vi "FLIM UI example.vi"(8 "error in (no error)":errorcluster) -> (0 "error out":errorcluster)   [LabVIEW 2014]
uses:
  typedefs/ScanControl_typedef.ctl
  typedefs/ScannerCommands_typedef.ctl
  typedefs/Command Queue element typedef.ctl
  SwabianInstruments.TimeTagger
panel:
  in  "Demo":bool caption="Enable demo signal"
  in  "Conditional Filter":bool
  in  "StopScan":bool
  out "Frame Progress":u8(slide) scale=0.0..100.0
  in  "scan_tagger":bool
  in  "TTs_found":i32(listbox)=-1 caption="Taggers found"
  out "Scanning":bool
  out "error msg":string caption="Error message"
  in  "Scan range":T1={"x-axis"={"start"=0.0, "num"=150, "step"=1.0}, "y-axis"={"start"=0.0, "num"=100, "step"=1.0}}
  out "Histogram at location":T2(graph)
  out "Intensity image":sgl[][](graph)
  in  "frame_start":enum32{"None", "Channel"}(tab) caption="Frame start marker"
  in  "FRAME_BEGIN_CH":i32
  in  "averages per frame":u32=1 min=1 step=1
  in  "frames to acquire":u32=1 step=1
  in  "n_bins":i32=100
  in  "Binwidth":dbl[unit]=1e-11
  in  "StartScan":bool
  in  "close":bool
  out "Time Tagger":string caption="Connected Time Tagger:"
  in  "Connect":bool
  in  "Pixel end marker":T3(tab)
  in  "Pixel duration time":dbl[unit] format="%^.3e"
  in  "PIXEL_END_CH":i32=-3
  in  "PIXEL_BEGIN_CH":i32=3
  in  "DET_CH":i32=2
  in  "LASER_CH":i32=1
  # "DESCRIPTION\nThis VI is an example.  It implements FLIM data acquisition part only and demonstrates how\nto use Flim class provided with the Time Tagger software.\n\nIt is designed as a template and a reasonybly good starting point for development of your \nown FLIM experiment control program.\n\nThis example provides demo signal that you can enable for testing purpose. The expected\nscan result with a demo sognal is a checkerboard-like intensity image."
  # "Do not use frame start marker.\nFrame begins automatcally."
  # "Pulse duration defines \npixel integration time"
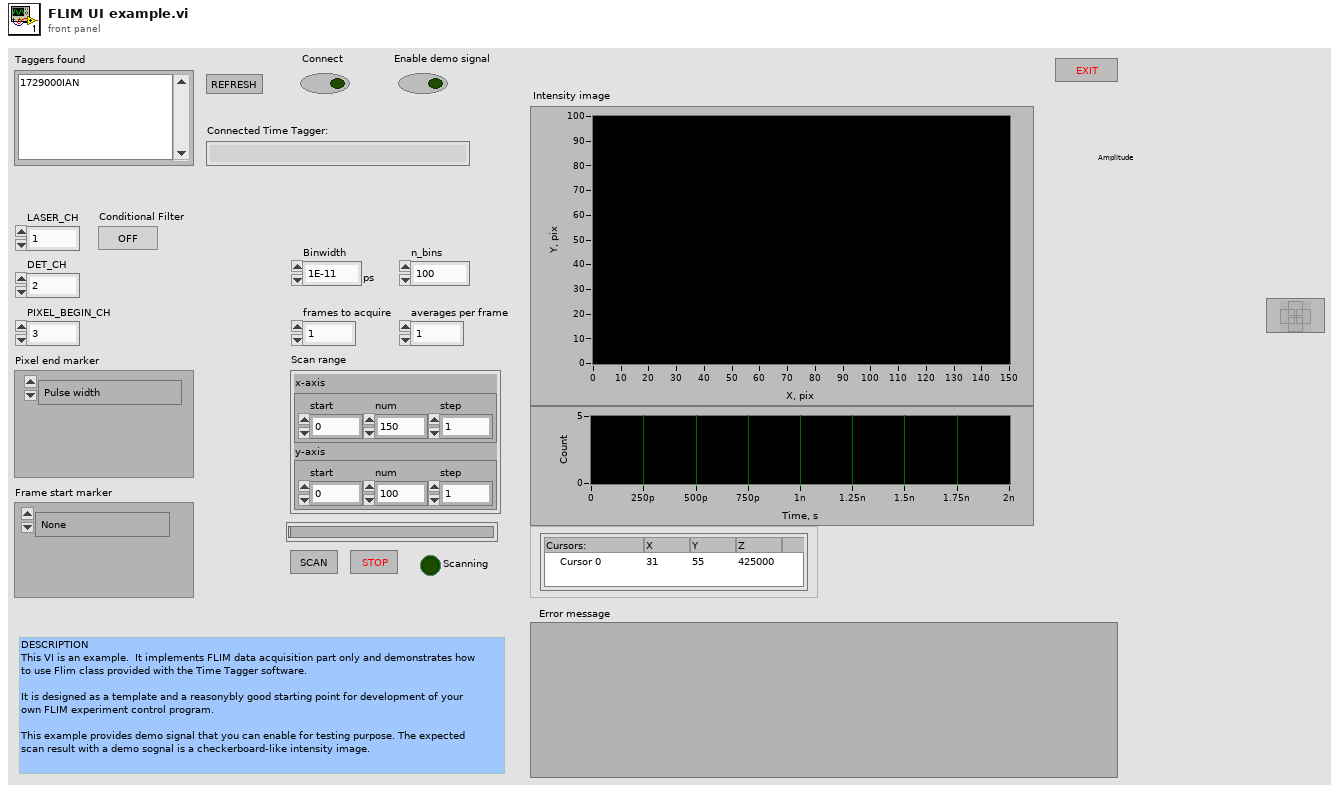
[diagram p1: front panel]
types:
  T1 = typedef "ScanControl_typedef.ctl" = cluster{"x-axis":cluster{"start":dbl, "num":u32, "step":dbl}, "y-axis":cluster{"start":dbl, "num":u32, "step":dbl}}
  T2 = cluster{dbl, "Binwidth":dbl[unit], "getHistograms":u32[]}
  T3 = enum32{"Pulse width", "Begin+duration", "End channel"}
  T4 = typedef "Command Queue element typedef.ctl" = cluster{"CMD":T5, "Scan range":T1}
  T5 = typedef "ScannerCommands_typedef.ctl" = enum16{"Do nothing", "Start Scan", "Stop Scan"}
  T6 = cluster{"TTlib":refnum<k24>, "tagger":refnum<k24>, "flim":refnum<k24>, "pixel_end_vch":refnum<k24>, "flim_frame":refnum<k24>, "Scan range":T1, "cmd_queue":refnum<queue>}
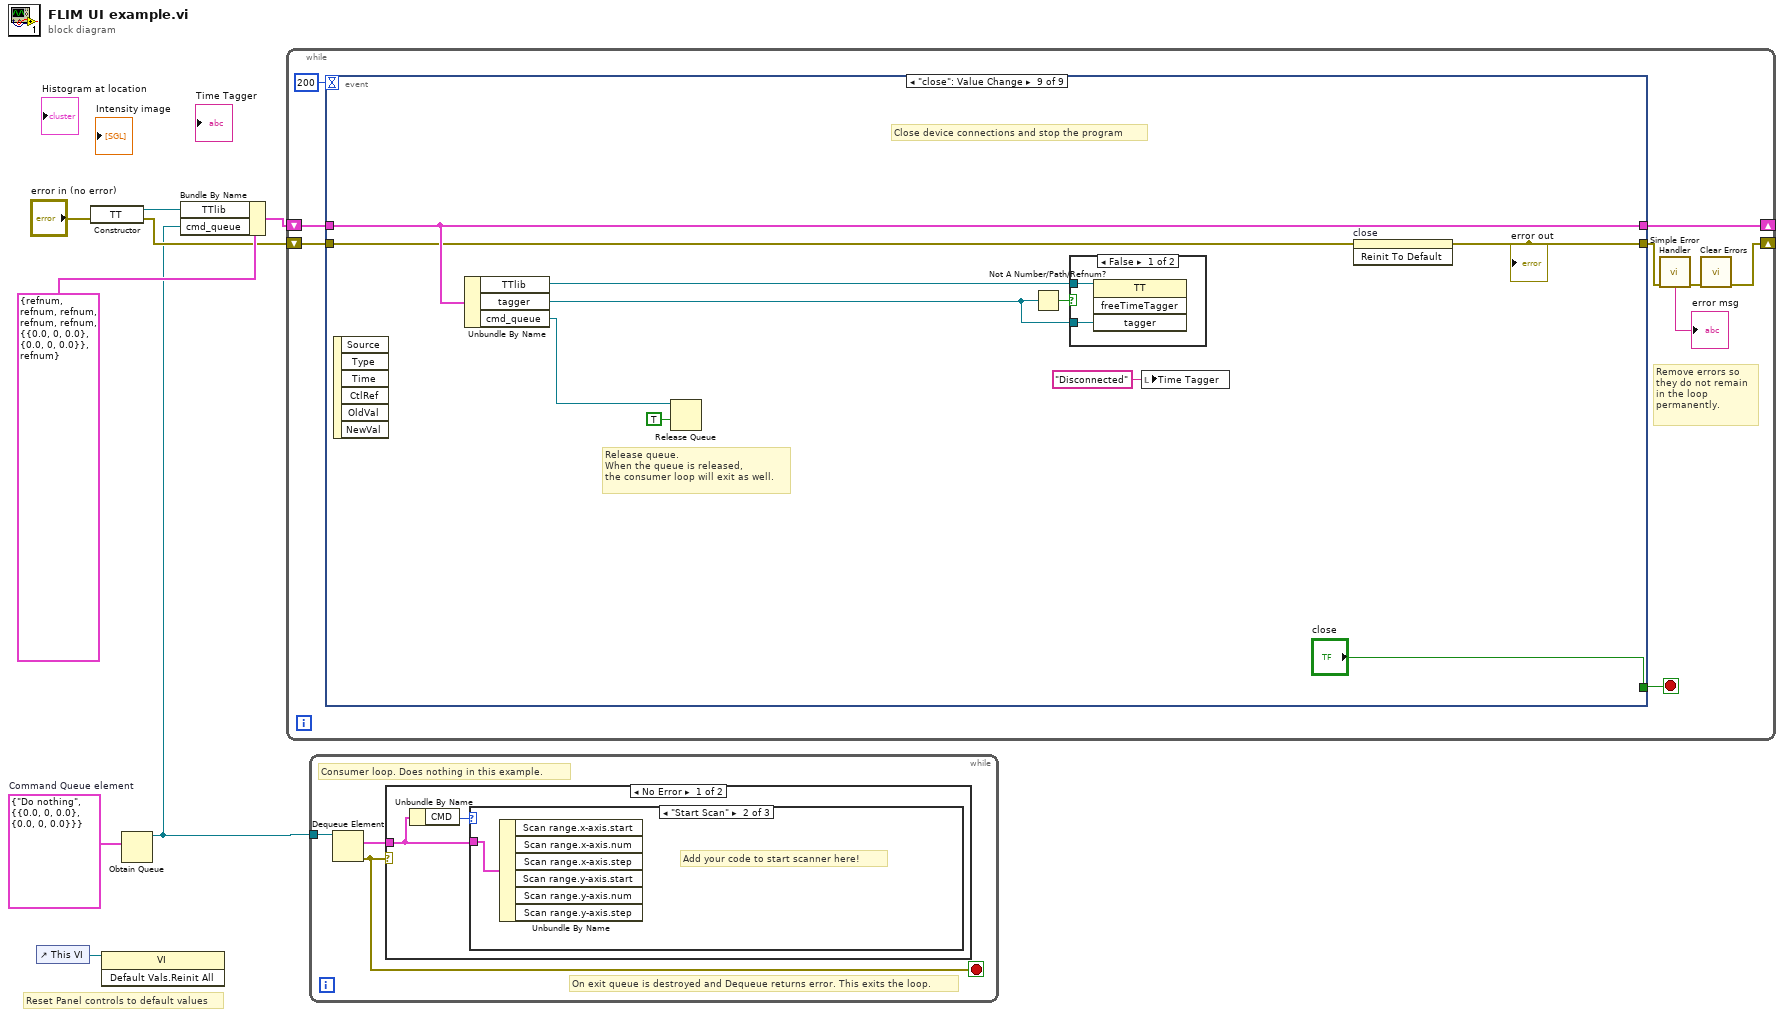
[diagram p0: block diagram]
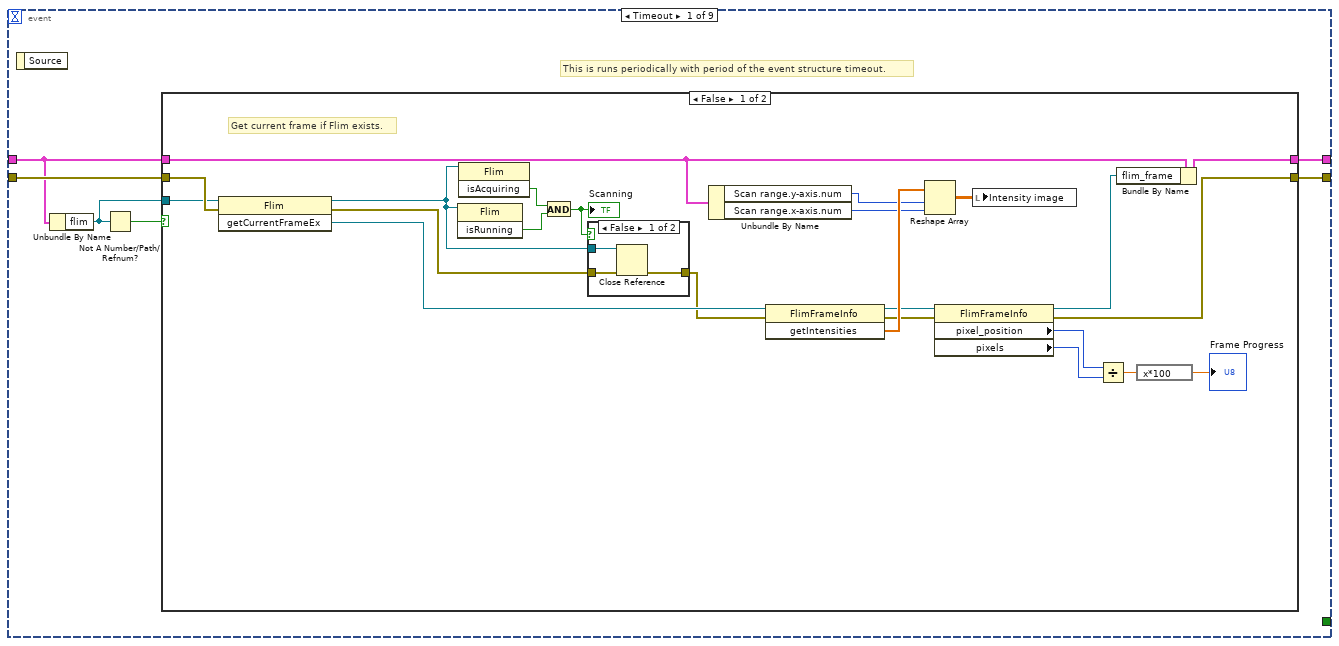
[diagram p5: hidden frame]
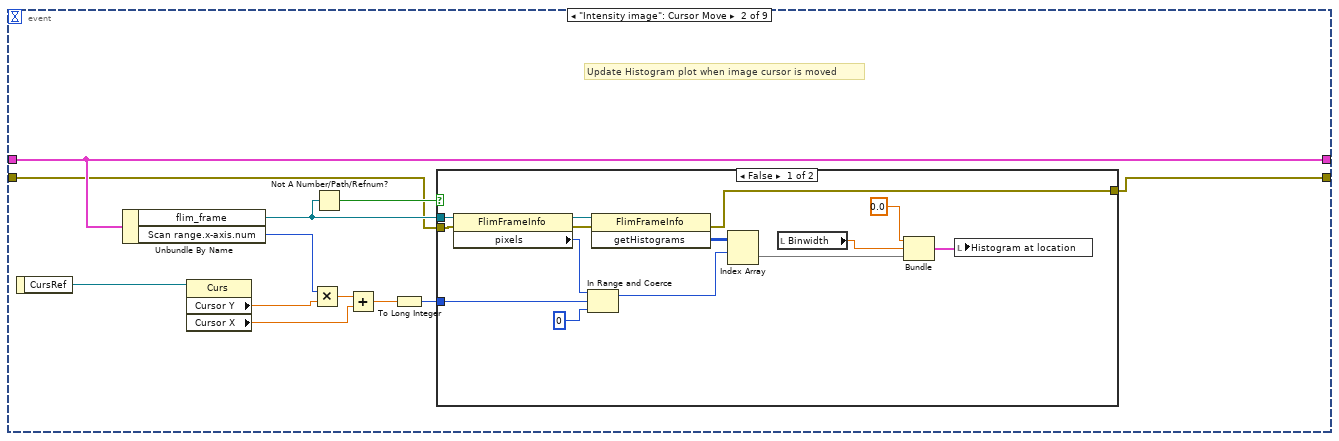
[diagram p8: hidden frame]
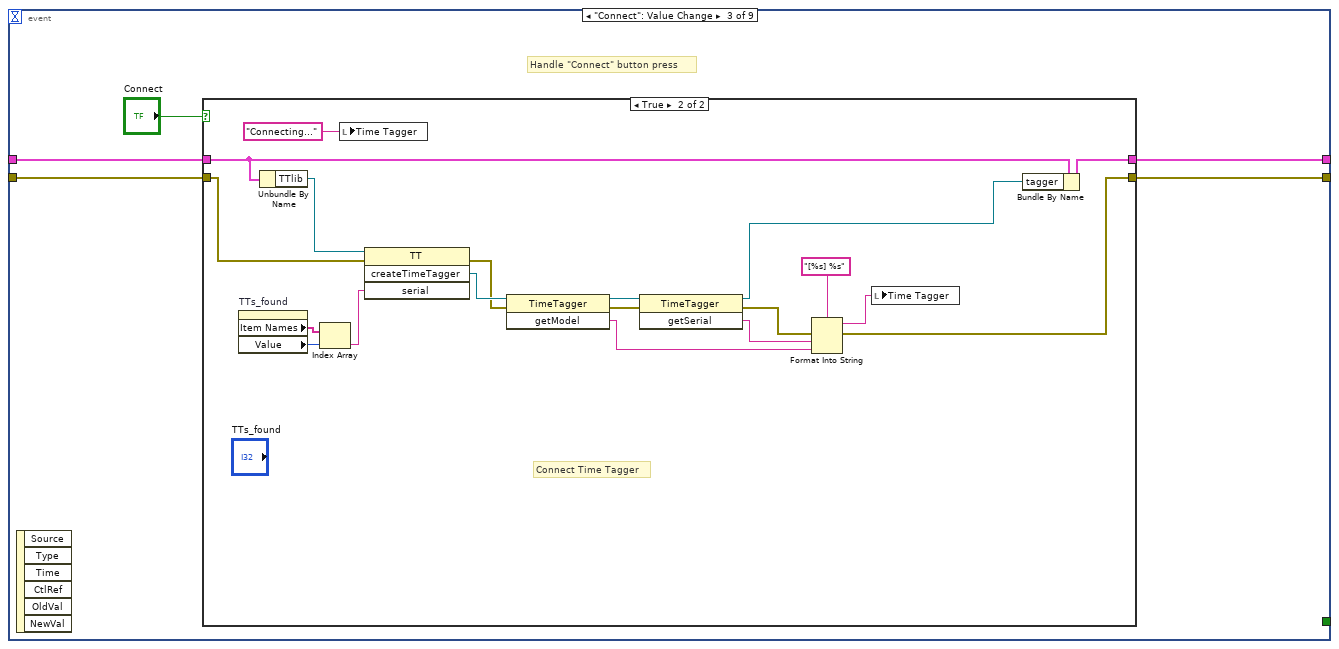
[diagram p10: hidden frame]
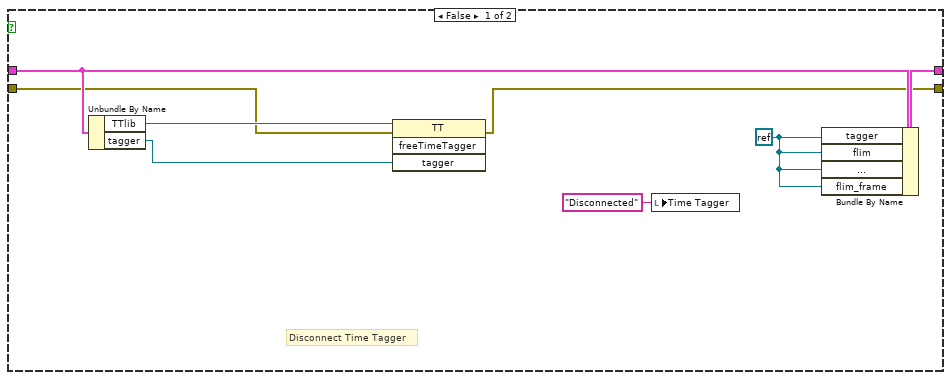
[diagram p11: hidden frame]
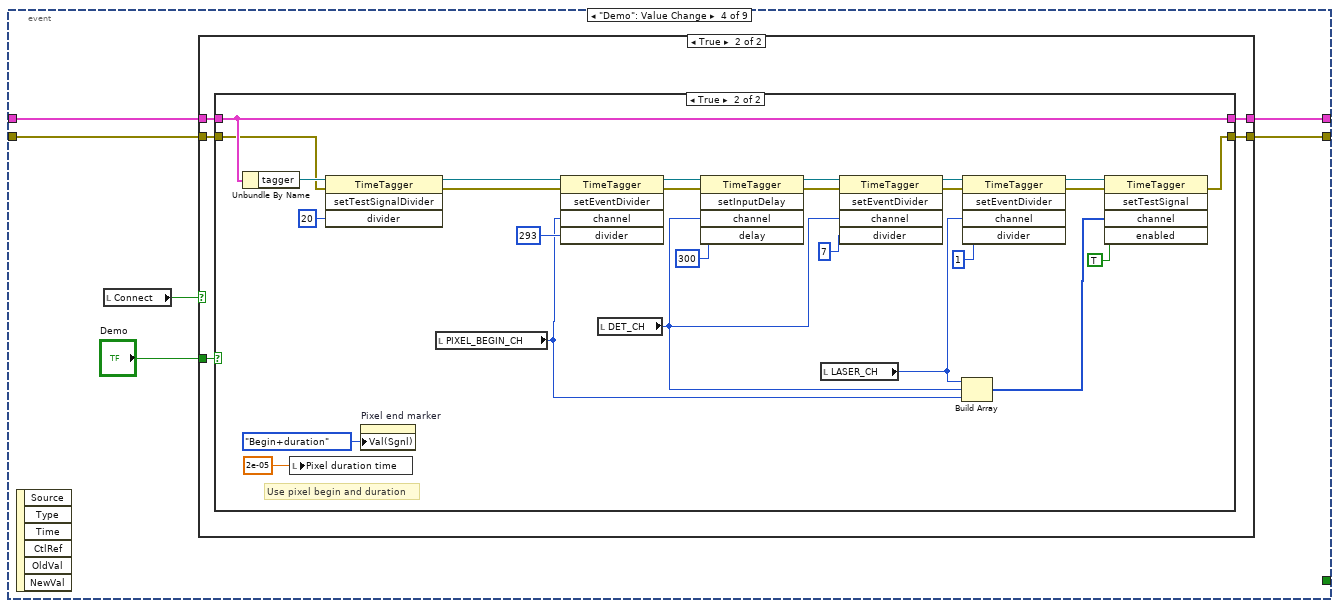
[diagram p12: hidden frame]
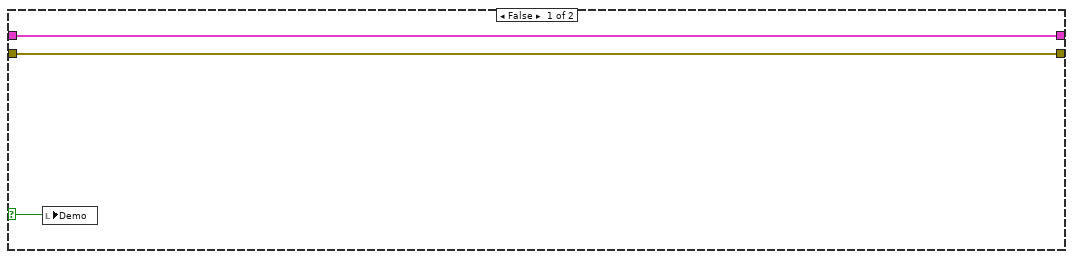
[diagram p13: hidden frame]
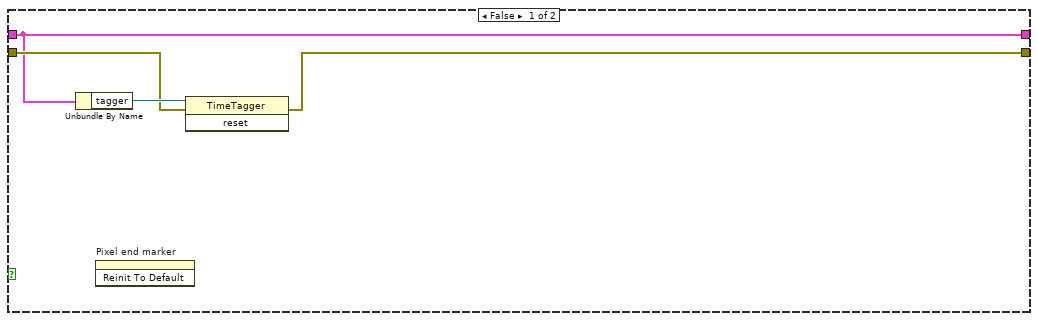
[diagram p14: hidden frame]
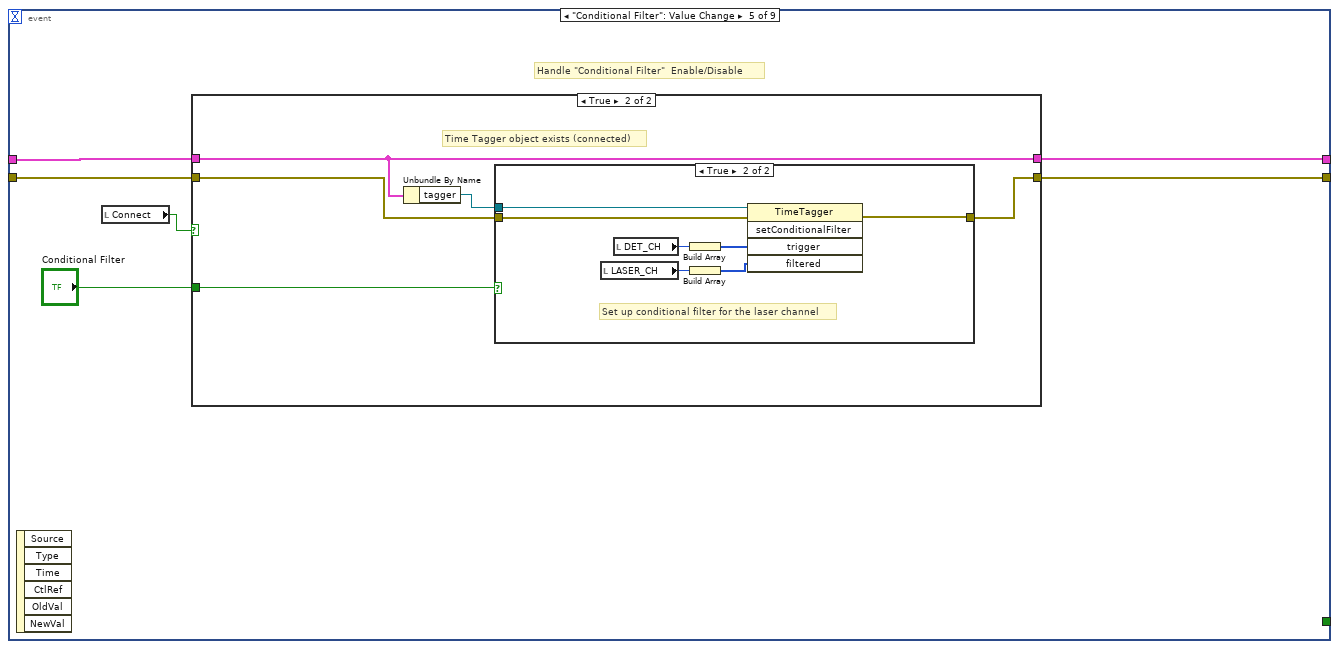
[diagram p15: hidden frame]
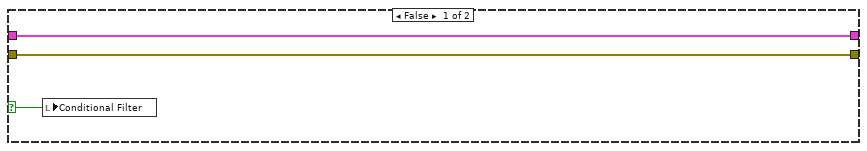
[diagram p16: hidden frame]
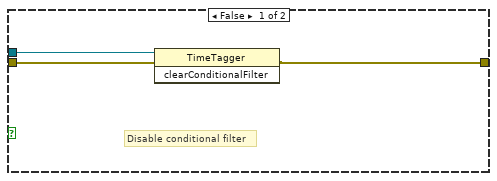
[diagram p17: hidden frame]
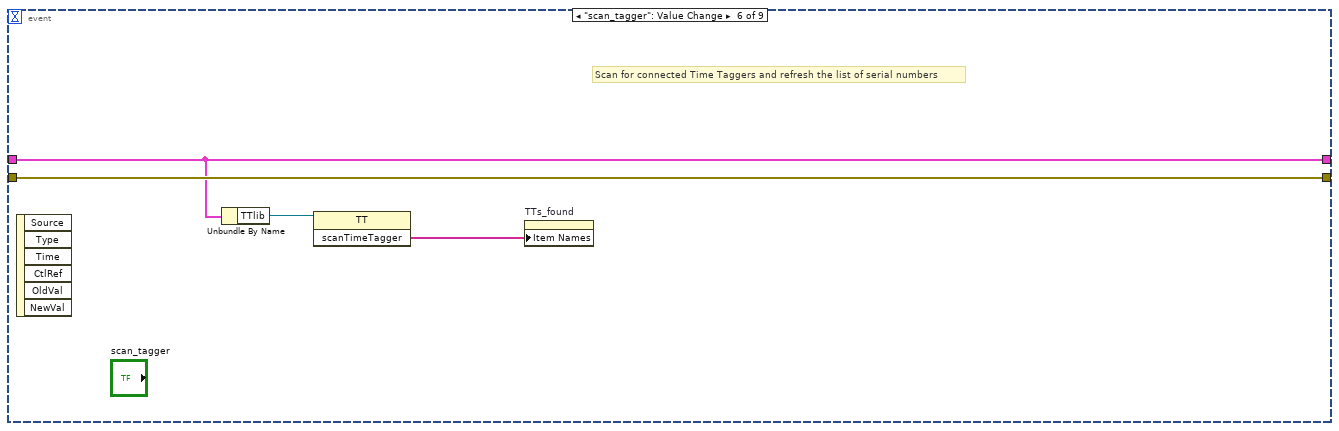
[diagram p18: hidden frame]
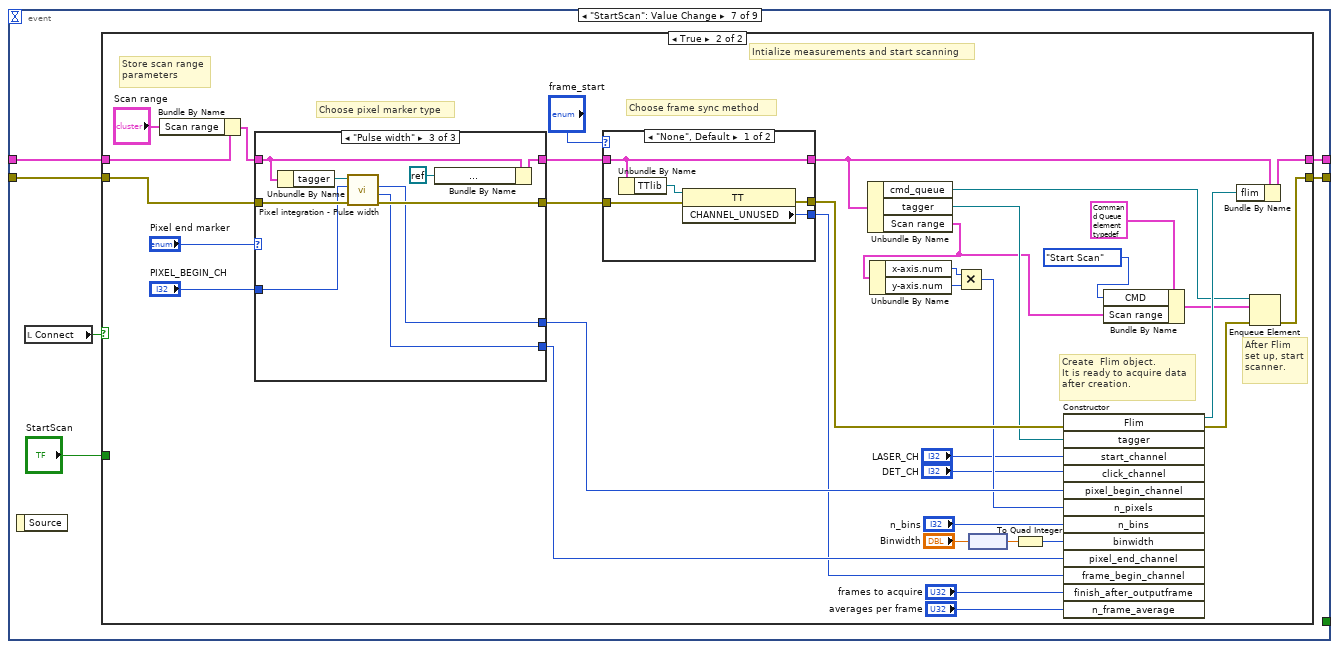
[diagram p19: hidden frame]
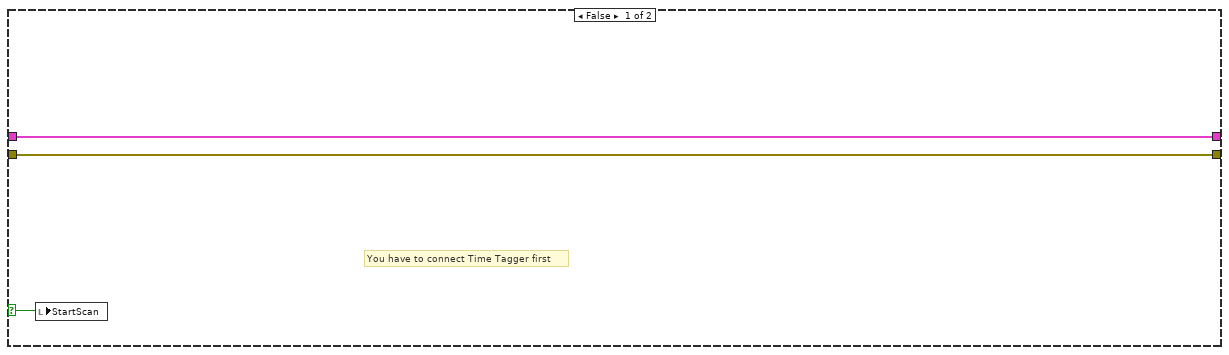
[diagram p20: hidden frame]
diagram:
  w4 = T4 {"CMD"=enum."Do nothing", "Scan range"={"x-axis"={"start"=0.0, "num"=0, "step"=0.0}, "y-axis"={"start"=0.0, "num"=0, "step"=0.0}}}  # Command Queue element
  # "Reset Panel controls to default values"
  n1 = control-ref of="This VI"() -> (w2:refnum<vi>)
  n2 = constructor class="TT"(error in="error in (no error)") -> (reference out=w6:refnum<k24>, error out=w5:errorcluster)  [unwired: 2 in, 1 out]
  n3 = invoke class="VI" method="Default Vals.Reinit All"(reference=w2) -> ()  [unwired: 2 in, 3 out]
  n4 = Obtain Queue(element data type=w4) -> (queue out=w3:refnum<queue>)  [unwired: 4 in, 2 out]
  n5 = Bundle By Name(cluster=T6 {"TTlib"=refnum, "tagger"=refnum, "flim"=refnum, "pixel_end_vch"=refnum, "flim_frame"=refnum, "Scan range"={"x-axis"={"start"=0.0, "num"=0, "step"=0.0}, "y-axis"={"start"=0.0, "num"=0, "step"=0.0}}, "cmd_queue"=refnum}, "TTlib"=w6, "cmd_queue"=w3) -> (w7:T6)
  n6 = while {
    shift-right: [w15] -> _
    shift-left: w7 -> [w16]
    shift-right: [w12] -> _
    shift-left: w5 -> [w14]
    stop <- w13 stop-if-true
    # "Remove errors so\nthey do not remain\nin the loop \npermanently."
    n7 = event shown="[8] \"close\": Value Change" {
      selector: _ -> [_ _ _ _ _ _ _ _ _]
      dyn-events: _ -> [_ _ _ _ _ _ _ _ _]
      timeout: 200 -> [_ _ _ _ _ _ _ _ _]
      tunnel: w16 -> [w22 w64 w84 w114 w158 w182 w189 w268 w281]
      tunnel: [w18 w64 w83 w115 w161 w182 w187 w268 w281] -> w15
      tunnel: w14 -> [w23 w58 w82 w112 w159 w183 w188 w269 w274]
      tunnel: [w19 w54 w81 w113 w160 w183 w186 w266 w273] -> w10
      tunnel: [_ _ _ _ _ _ _ _ "close"] -> w13
      event Timeout {
        # "This is runs periodically with period of the event structure timeout."
        n8 = event-data() -> ()  [unwired: 1 in, 1 out]
        n9 = Unbundle By Name(w22) -> ("flim"=w20:refnum<k24>)
        n10 = Not A Number/Path/Refnum?(number/path/refnum=w20) -> (NaN/Path/Refnum?=w21:bool)
        n11 = case shown="False" w21 {
          tunnel: w22 -> [w31 w52]
          tunnel: w23 -> [w46 w51]
          tunnel: [w25 w52] -> w18
          tunnel: [w30 w51] -> w19
          tunnel: w20 -> [w45 _]
          frame False {
            # "Get current frame if Flim exists."
            n12 = invoke class="Flim" method="getCurrentFrameEx"(reference=w45, error in=w46) -> (reference out=w27:refnum<k24>, error out=w29:errorcluster, "getCurrentFrameEx"=w42:refnum<k24>)  [unwired: 1 in]
            n13 = invoke class="Flim" method="isRunning"(reference=w27) -> ("isRunning"=w43:bool)  [unwired: 2 in, 2 out]
            n14 = invoke class="Flim" method="isAcquiring"(reference=w27) -> ("isAcquiring"=w44:bool)  [unwired: 2 in, 2 out]
            n15 = And(x=w44, y=w43) -> (x .and. y?=w26:bool)
            "Scanning" <- w26
            n16 = case shown="False" w26 {
              tunnel: w29 -> [w49 w50]
              tunnel: [w48 w50] -> w28
              tunnel: w27 -> [w47 _]
              frame False {
                n17 = Close Reference(reference=w47, error in (no error)=w49) -> (error out=w48:errorcluster)
              }
              frame True {
              }
            }
            n18 = Unbundle By Name(w31) -> ("Scan range.y-axis.num"=w39:u32, "Scan range.x-axis.num"=w38:u32)
            n19 = invoke class="FlimFrameInfo" method="getIntensities"(reference=w42, error in=w28) -> (reference out=w36:refnum<k24>, error out=w37:errorcluster, "getIntensities"=w40:sgl[])  [unwired: 1 in]
            n20 = Reshape Array(w40, w39, w38) -> (w41:sgl[][])
            n21 = property class="FlimFrameInfo"(reference=w36, error in=w37) -> (reference out=w24:refnum<k24>, error out=w30:errorcluster, "pixel_position"=w34:u32, "pixels"=w35:u32)
            n22 = local write "Intensity image"(w41) -> ()
            n23 = Divide(x=w34, y=w35) -> (x/y=w33:dbl)
            n24 = Bundle By Name(cluster=w31, "flim_frame"=w24) -> (w25:T6)
            n25 = expression code="x*100"(w33) -> (→"Frame Progress":dbl)
          }
          frame True {
            # "Flim instance does not exist.\nHave you started the scan?"
          }
        }
      }
      event "Intensity image": Cursor Move {
        # "Update Histogram plot when image cursor is moved"
        n26 = event-data() -> ("CursRef"=w55:refnum<vi>)  [unwired: 1 in]
        n27 = Unbundle By Name(w64) -> ("flim_frame"=w59:refnum<k24>, "Scan range.x-axis.num"=w63:u32)
        n28 = property class="Curs"(reference=w55) -> ("Cursor Y"=w57:dbl, "Cursor X"=w56:dbl)  [unwired: 1 in, 2 out]
        n29 = Multiply(x=w63, y=w57) -> (x*y=w62:dbl)
        n30 = Not A Number/Path/Refnum?(number/path/refnum=w59) -> (NaN/Path/Refnum?=w60:bool)
        n31 = Add(x=w62, y=w56) -> (x+y=w61:dbl)
        n32 = To Long Integer(number=w61) -> (32bit integer=w53:i32)
        n33 = case shown="False" w60 {
          tunnel: w59 -> [w73 _]
          tunnel: w53 -> [w70 _]
          tunnel: w58 -> [w68 w79]
          tunnel: [w65 w79] -> w54
          frame False {
            n34 = property class="FlimFrameInfo"(reference=w73, error in=w68) -> (reference out=w72:refnum<k24>, error out=w67:errorcluster, "pixels"=w71:u32)
            n35 = In Range and Coerce(upper limit=w71, x=w70, lower limit=u32 0) -> (coerced(x)=w66:u32)  [unwired: 1 out]
            n36 = invoke class="FlimFrameInfo" method="getHistograms"(reference=w72, error in=w67) -> (error out=w65:errorcluster, "getHistograms"=w78:u32[][])  [unwired: 1 in, 1 out]
            n37 = Index Array(array=w78, index (row)=w66) -> (element=w77:u32[])  [unwired: 1 in]
            n38 = local read "Binwidth"() -> (w76:dbl[unit])
            n39 = Bundle(0.0, "Binwidth"=w76, "getHistograms"=w77) -> (w74:T2)  [unwired: 1 in]
            n40 = local write "Histogram at location"(w74) -> ()
          }
          frame True {
          }
        }
      }
      event "Connect": Value Change {
        # "Handle \"Connect\" button press"
        n41 = event-data() -> ()  [unwired: 1 in, 6 out]
        n42 = case shown="True" "Connect" {
          tunnel: w84 -> [w92 w109]
          tunnel: [w91 w110] -> w83
          tunnel: w82 -> [w88 w111]
          tunnel: [w87 w106] -> w81
          frame False {
            w85 = refnum<k0> refnum
            # "Disconnect Time Tagger"
            n43 = Unbundle By Name(w92) -> ("TTlib"=w90:refnum<k24>, "tagger"=w89:refnum<k24>)
            n44 = invoke class="TT" method="freeTimeTagger"(reference=w90, error in=w88, "tagger"=w89) -> (error out=w87:errorcluster)  [unwired: 1 in, 3 out]
            n45 = local write "Time Tagger"("Disconnected" ("Time Tagger")) -> ()
            n46 = Bundle By Name(cluster=w92, "tagger"=w85, "flim"=w85, "pixel_end_vch"=w85, "flim_frame"=w85) -> (w91:T6)
          }
          frame True {
            # "Connect Time Tagger"
            n47 = property on="TTs_found" class="LstBox (strict)"() -> ("Item Names"=w96:string[], "Value"=w95:i32)  [unwired: 2 in, 2 out]
            n48 = Unbundle By Name(w109) -> ("TTlib"=w108:refnum<k24>)
            n49 = Index Array(array=w96, index=w95) -> (element=w94:string)
            n50 = local write "Time Tagger"("Connecting..." ("Time Tagger")) -> ()
            n51 = invoke class="TT" method="createTimeTagger"(reference=w108, error in=w111, "serial"=w94) -> (error out=w104:errorcluster, "createTimeTagger"=w105:refnum<k24>)  [unwired: 1 in, 2 out]
            n52 = invoke class="TimeTagger" method="getModel"(reference=w105, error in=w104) -> (reference out=w102:refnum<k24>, error out=w103:errorcluster, "getModel"=w97:string)  [unwired: 1 in]
            n53 = invoke class="TimeTagger" method="getSerial"(reference=w102, error in=w103) -> (reference out=w107:refnum<k24>, error out=w100:errorcluster, "getSerial"=w98:string)  [unwired: 1 in]
            n54 = Format Into String(format string="[%s] %s", error in=w100, w98, w97) -> (resulting string=w101:string, error out=w106:errorcluster)  [unwired: 1 in]
            n55 = local write "Time Tagger"(w101) -> ()
            n56 = Bundle By Name(cluster=w109, "tagger"=w107) -> (w110:T6)
          }
        }
      }
      event "Demo": Value Change {
        n57 = event-data() -> ()  [unwired: 1 in, 6 out]
        n58 = local read "Connect"() -> (w117:bool)
        n59 = case shown="True" w117 {
          selector: w117 -> [w120 _]
          tunnel: "Demo" -> [_ w124]
          tunnel: [w118 w121] -> w115
          tunnel: w114 -> [w118 w125]
          tunnel: [w119 w122] -> w113
          tunnel: w112 -> [w119 w123]
          frame False {
            n60 = local write "Demo"(w120) -> ()
          }
          frame True {
            n61 = case shown="True" w124 {
              tunnel: w125 -> [w126 w154]
              tunnel: w123 -> [w128 w134]
              tunnel: [w127 w143] -> w122
              tunnel: [w126 w154] -> w121
              frame False {
                n62 = Unbundle By Name(w126) -> ("tagger"=w129:refnum<k24>)
                n63 = invoke on="Pixel end marker" class="TabCtl (strict)" method="Reinit To Default"() -> ()  [unwired: 3 in, 3 out]
                n64 = invoke class="TimeTagger" method="reset"(reference=w129, error in=w128) -> (error out=w127:errorcluster)  [unwired: 1 in, 2 out]
              }
              frame True {
                # "Use pixel begin and duration"
                n65 = Unbundle By Name(w154) -> ("tagger"=w155:refnum<k24>)
                n66 = local write "Pixel duration time"(dbl[unit] 2e-05 ("Pixel duration time")) -> ()
                n67 = invoke class="TimeTagger" method="setTestSignalDivider"(reference=w155, error in=w134, "divider"=20) -> (reference out=w135:refnum<k24>, error out=w133:errorcluster)  [unwired: 1 in, 2 out]
                n68 = property on="Pixel end marker" class="TabCtl (strict)"("Val(Sgnl)"=T3."Begin+duration" ("Value (Signaling)")) -> ()  [unwired: 2 in, 2 out]
                n69 = local read "PIXEL_BEGIN_CH"() -> (w148:i32)
                n70 = invoke class="TimeTagger" method="setEventDivider"(reference=w135, error in=w133, "channel"=w148, "divider"=u32 293) -> (reference out=w152:refnum<k24>, error out=w151:errorcluster)  [unwired: 1 in, 3 out]
                n71 = local read "DET_CH"() -> (w145:i32)
                n72 = invoke class="TimeTagger" method="setInputDelay"(reference=w152, error in=w151, "channel"=w145, "delay"=i64 300) -> (reference out=w146:refnum<k24>, error out=w142:errorcluster)  [unwired: 1 in, 3 out]
                n73 = local read "LASER_CH"() -> (w140:i32)
                n74 = invoke class="TimeTagger" method="setEventDivider"(reference=w146, error in=w142, "channel"=w145, "divider"=u32 7) -> (reference out=w137:refnum<k24>, error out=w138:errorcluster)  [unwired: 1 in, 3 out]
                n75 = Build Array(w140, w145, w148) -> (w147:i32[])
                n76 = invoke class="TimeTagger" method="setEventDivider"(reference=w137, error in=w138, "channel"=w140, "divider"=u32 1) -> (reference out=w141:refnum<k24>, error out=w136:errorcluster)  [unwired: 1 in, 3 out]
                n77 = invoke class="TimeTagger" method="setTestSignal"(reference=w141, error in=w136, "channel"=w147, "enabled"=TRUE) -> (error out=w143:errorcluster)  [unwired: 1 in, 4 out]
              }
            }
          }
        }
      }
      event "Conditional Filter": Value Change {
        # "Handle \"Conditional Filter\"  Enable/Disable"
        n78 = event-data() -> ()  [unwired: 1 in, 6 out]
        n79 = local read "Connect"() -> (w156:bool)
        n80 = case shown="True" w156 {
          selector: w156 -> [w162 _]
          tunnel: [w164 w166] -> w161
          tunnel: w158 -> [w164 w166]
          tunnel: [w163 w167] -> w160
          tunnel: w159 -> [w163 w168]
          tunnel: "Conditional Filter" -> [_ w169]
          frame False {
            n81 = local write "Conditional Filter"(w162) -> ()
          }
          frame True {
            # "Time Tagger object exists (connected)"
            n82 = Unbundle By Name(w166) -> ("tagger"=w165:refnum<k24>)
            n83 = case shown="True" w169 {
              tunnel: w165 -> [w172 w179]
              tunnel: w168 -> [w171 w174]
              tunnel: [w170 w173] -> w167
              frame False {
                # "Disable conditional filter"
                n84 = invoke class="TimeTagger" method="clearConditionalFilter"(reference=w172, error in=w171) -> (error out=w170:errorcluster)  [unwired: 1 in, 2 out]
              }
              frame True {
                # "Set up conditional filter for the laser channel"
                n85 = local read "LASER_CH"() -> (w175:i32)
                n86 = local read "DET_CH"() -> (w176:i32)
                n87 = Build Array(w176) -> (w178:i32[])
                n88 = Build Array(w175) -> (w177:i32[])
                n89 = invoke class="TimeTagger" method="setConditionalFilter"(reference=w179, error in=w174, "trigger"=w178, "filtered"=w177) -> (error out=w173:errorcluster)  [unwired: 1 in, 4 out]
              }
            }
          }
        }
      }
      event "scan_tagger": Value Change {
        # "Scan for connected Time Taggers and refresh the list of serial numbers"
        n90 = event-data() -> ()  [unwired: 1 in, 6 out]
        n91 = Unbundle By Name(w182) -> ("TTlib"=w180:refnum<k24>)
        n92 = invoke class="TT" method="scanTimeTagger"(reference=w180) -> ("scanTimeTagger"=w181:string[])  [unwired: 2 in, 2 out]
        n93 = property on="TTs_found" class="LstBox (strict)"("Item Names"=w181) -> ()  [unwired: 2 in, 2 out]
      }
      event "StartScan": Value Change {
        n94 = event-data() -> ()  [unwired: 1 in, 1 out]
        n95 = local read "Connect"() -> (w184:bool)
        n96 = case shown="True" w184 {
          selector: w184 -> [w191 _]
          tunnel: w189 -> [w192 w227]
          tunnel: w188 -> [w190 w226]
          tunnel: [w192 w225] -> w187
          tunnel: [w190 w200] -> w186
          tunnel: "StartScan" -> [_ _]
          frame False {
            # "You have to connect Time Tagger first"
            n97 = local write "StartScan"(w191) -> ()
          }
          frame True {
            # "Intialize measurements and start scanning"
            # "Store scan range\nparameters"
            # "Choose pixel marker type"
            # "Choose frame sync method"
            # "Create  Flim object.\nIt is ready to acquire data\nafter creation."
            # "After Flim\nset up, start\nscanner."
            n98 = Bundle By Name(cluster=w227, "Scan range"="Scan range") -> (w203:T6)
            n99 = case shown="\"Pulse width\"" "Pixel end marker" {
              tunnel: "PIXEL_BEGIN_CH" -> [w241 w249 w257]
              tunnel: [w245 w253 w254] -> w216
              tunnel: w203 -> [w244 w252 w255]
              tunnel: [w239 w249 w259] -> w218
              tunnel: [w238 "PIXEL_END_CH" w260] -> w217
              tunnel: w226 -> [w237 w248 w262]
              tunnel: [w236 w248 w261] -> w215
              frame "Begin+duration", Default {
                n100 = Unbundle By Name(w244) -> ("tagger"=w243:refnum<k24>)
                n101 = node("Pixel duration time") -> (w246:dbl)
                n102 = To Quad Integer(1:w246) -> (0:w240:i64)
                n103 = call "Pixel integration - Pixel begin and duration.vi"("error in (no error)"=w237, "duration, (ps)"=w240, "pixel_start_ch"=w241, "tagger in"=w243) -> ("error out"=w236:errorcluster, "pixel_end_ch"=w238:i32, "pixel_start_ch"=w239:i32, "delayed channel out"=w242:refnum<k24>)  [unwired: 4 in]
                n104 = Bundle By Name(cluster=w244, "pixel_end_vch"=w242) -> (w245:T6)
              }
              frame "End channel" {
                n105 = Bundle By Name(cluster=w252, "pixel_end_vch"=refnum<k0> refnum) -> (w253:T6)
              }
              frame "Pulse width" {
                n106 = Unbundle By Name(w255) -> ("tagger"=w258:refnum<k24>)
                n107 = call "Pixel integration - Pulse width.vi"("error in (no error)"=w262, "channel"=w257, "tagger in"=w258) -> ("error out"=w261:errorcluster, "pixel_end_ch"=w260:i32, "pixel_start_ch"=w259:i32)  [unwired: 6 in]
                n108 = Bundle By Name(cluster=w255, "pixel_end_vch"=refnum<k0> refnum) -> (w254:T6)
              }
            }
            n109 = case shown="\"None\", Default" "frame_start" {
              tunnel: [w231 "FRAME_BEGIN_CH"] -> w210
              tunnel: w216 -> [w230 w234]
              tunnel: [w230 w234] -> w212
              tunnel: w215 -> [w229 w233]
              tunnel: [w228 w233] -> w214
              frame "None", Default {
                n110 = Unbundle By Name(w230) -> ("TTlib"=w232:refnum<k24>)
                n111 = property class="TT"(reference=w232, error in=w229) -> (error out=w228:errorcluster, "CHANNEL_UNUSED"=w231:i32)  [unwired: 1 out]
              }
              frame "Channel" {
              }
            }
            n112 = Unbundle By Name(w212) -> ("cmd_queue"=w199:refnum<queue>, "tagger"=w213:refnum<k24>, "Scan range"=w196:T1)
            n113 = Unbundle By Name(w196) -> ("x-axis.num"=w206:u32, "y-axis.num"=w205:u32)
            n114 = Multiply(x=w206, y=w205) -> (x*y=w204:u32)
            n115 = node("Binwidth") -> (w221:dbl)
            n116 = To Quad Integer(1:w221) -> (0:w223:i64)
            n117 = constructor class="Flim"(error in=w214, "tagger"=w213, "start_channel"="LASER_CH", "click_channel"="DET_CH", "pixel_begin_channel"=w218, "n_pixels"=w204, "n_bins"="n_bins", "binwidth"=w223, "pixel_end_channel"=w217, "frame_begin_channel"=w210, "finish_after_outputframe"="frames to acquire", "n_frame_average"="averages per frame") -> (reference out=w211:refnum<k24>, error out=w201:errorcluster)  [unwired: 2 in, 12 out]
            n118 = Bundle By Name(cluster=T4 {"CMD"=enum."Do nothing", "Scan range"={"x-axis"={"start"=0.0, "num"=0, "step"=0.0}, "y-axis"={"start"=0.0, "num"=0, "step"=0.0}}} ("Cluster"), "CMD"=ScannerCommands_typedef."Start Scan", "Scan range"=w196) -> (w197:T4)
            n119 = Bundle By Name(cluster=w212, "flim"=w211) -> (w225:T6)
            n120 = Enqueue Element(queue=w199, element=w197, error in (no error)=w201) -> (error out=w200:errorcluster)  [unwired: 1 in, 2 out]
          }
        }
      }
      event "StopScan": Value Change {
        # "Interrupt scanning"
        # "Stop Flim class if exists"
        n121 = event-data() -> ()  [unwired: 1 in, 6 out]
        n122 = Unbundle By Name(w268) -> ("flim"=w270:refnum<k24>, "cmd_queue"=w267:refnum<queue>)
        n123 = Bundle By Name(cluster=T4 {"CMD"=enum."Stop Scan", "Scan range"={"x-axis"={"start"=0.0, "num"=0, "step"=0.0}, "y-axis"={"start"=0.0, "num"=0, "step"=0.0}}} ("Cluster"), "CMD"=ScannerCommands_typedef."Stop Scan") -> (w264:T4)
        n124 = Enqueue Element(queue=w267, element=w264, error in (no error)=w269) -> (error out=w266:errorcluster)  [unwired: 1 in, 2 out]
        n125 = Not A Number/Path/Refnum?(number/path/refnum=w270) -> (NaN/Path/Refnum?=w271:bool)
        n126 = case shown="False" w271 {
          tunnel: w270 -> [w272 _]
          frame False {
            n127 = invoke class="Flim" method="stop"(reference=w272) -> ()  [unwired: 2 in, 3 out]
          }
          frame True {
          }
        }
      }
      event "close": Value Change {
        # "Close device connections and stop the program"
        # "Release queue.\nWhen the queue is released, \nthe consumer loop will exit as well."
        n128 = event-data() -> ()  [unwired: 1 in, 6 out]
        n129 = Unbundle By Name(w281) -> ("TTlib"=w280:refnum<k24>, "tagger"=w279:refnum<k24>, "cmd_queue"=w275:refnum<queue>)
        n130 = Release Queue(queue=w275, force destroy? (F)=TRUE) -> ()  [unwired: 1 in, 3 out]
        n131 = Not A Number/Path/Refnum?(number/path/refnum=w279) -> (NaN/Path/Refnum?=w278:bool)
        n132 = case shown="False" w278 {
          tunnel: w280 -> [w284 _]
          tunnel: w279 -> [w283 _]
          frame False {
            n133 = invoke class="TT" method="freeTimeTagger"(reference=w284, "tagger"=w283) -> ()  [unwired: 2 in, 4 out]
          }
          frame True {
          }
        }
        n134 = local write "Time Tagger"("Disconnected" ("Time Tagger")) -> ()
        n135 = invoke on="close" class="Bool (strict)" method="Reinit To Default"(error in=w274) -> (error out=w273:errorcluster)  [unwired: 2 in, 2 out]
        "error out" <- w273
      }
    }
    n136 = call <vilib>:"Simple Error Handler.vi"("error in (no error)"=w10) -> ("error out"=w11:errorcluster, "message"=→"error msg":string)  [unwired: 4 in, 3 out]
    n137 = call <vilib>:"Clear Errors.vi"("error in (no error)"=w11) -> ("error out"=w12:errorcluster)  [unwired: 5 in, 1 out]
  }
  n138 = while {
    tunnel: w3 -> [w287]
    stop <- w285 stop-if-true
    # "On exit queue is destroyed and Dequeue returns error. This exits the loop."
    # "Consumer loop. Does nothing in this example."
    n139 = Dequeue Element(queue=w287) -> (element=w286:T4, error out=w285:errorcluster)  [unwired: 2 in, 2 out]
    n140 = case shown="No Error" w285 {
      tunnel: w286 -> [w288 _]
      frame No Error {
        n141 = Unbundle By Name(w288) -> ("CMD"=w289:T5)
        n142 = case shown="\"Start Scan\"" w289 {
          tunnel: w288 -> [_ w290 _]
          frame "Do nothing" {
            # "This is a placeholder state that shall have no operation"
          }
          frame "Start Scan" {
            # "Add your code to start scanner here!"
            n143 = Unbundle By Name(w290) -> ()  [unwired: 6 out]
          }
          frame "Stop Scan" {
            # "Add your code to stop"
          }
        }
      }
      frame Error {
      }
    }
  }
